vi "Aggiorna colori caselle VACON.vi"(7 "id":i32, 10 "Letture inverter":T1, 11 "Test settings":refnum<vi>) -> ()   [LabVIEW 2019]
uses:
  Letture inverter.ctl
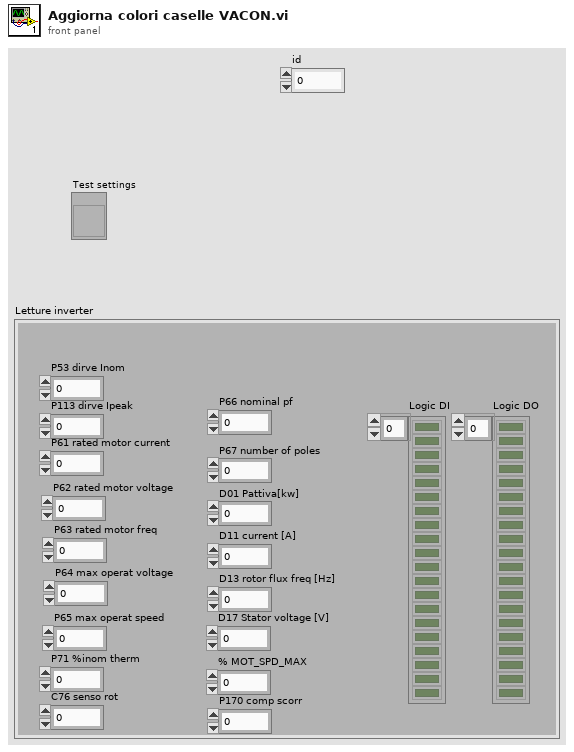
[diagram p1: front panel]
types:
  T1 = typedef "Letture inverter.ctl" = cluster{"P61 rated motor current":dbl, "P62 rated motor voltage":dbl, "P63 rated motor freq":dbl, "P64 max operat voltage":dbl, "P65 max operat speed":dbl, "P66 nominal pf":dbl, "P67 number of poles":dbl, "D01 Pattiva[kw]":dbl, "D11 current [A]":dbl, "D13 rotor flux freq [Hz]":dbl, "D17 Stator voltage [V]":dbl, "% MOT_SPD_MAX":dbl, "Logic DI":bool[], "Logic DO":bool[], "P71 %inom therm":dbl, "P53 dirve Inom":dbl, "P113 dirve Ipeak":dbl, "C76 senso rot":dbl, "P170 comp scorr":dbl}
  T2 = typedef "Parametri inverter.ctl" = cluster{"Vn [V]":dbl, "Fn [Hz]":dbl, "CosFi":dbl, "Imax [%Inom]":dbl, "#poles":dbl, "Inom [A]":dbl, "Senso rotazione":enum16{"CW", "CCW"}, "RPM nom":dbl, "Fmax[Hz]":dbl}
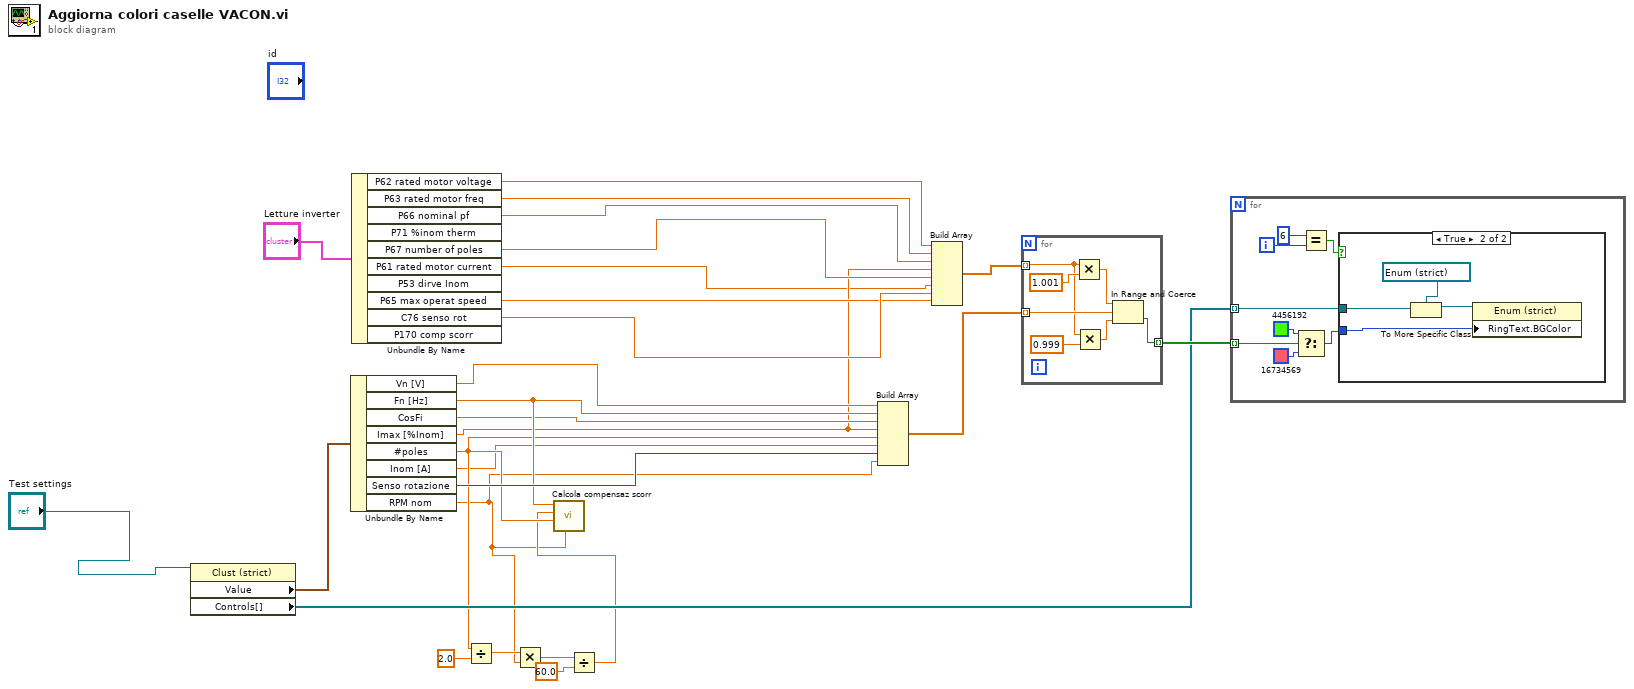
[diagram p0: block diagram]
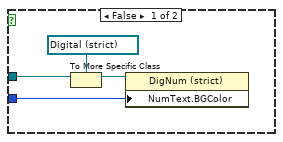
[diagram p2: hidden frame]
diagram:
  n1 = property class="Clust (strict)"(reference="Test settings") -> ("Value"=w21:T2, "Controls[]"=w22:refnum<vi>[])  [unwired: 1 in, 2 out]
  n2 = Unbundle By Name(w21) -> ("Vn [V]"=w5:dbl, "Fn [Hz]"=w16:dbl, "CosFi"=w15:dbl, "Imax [%Inom]"=w4:dbl, "#poles"=w10:dbl, "Inom [A]"=w2:dbl, "Senso rotazione"=w17:enum16{"CW", "CCW"}, "RPM nom"=w7:dbl)
  n3 = Unbundle By Name("Letture inverter") -> ("P62 rated motor voltage"=w26:dbl, "P63 rated motor freq"=w25:dbl, "P66 nominal pf"=w8:dbl, "P67 number of poles"=w24:dbl, "P61 rated motor current"=w3:dbl, "P65 max operat speed"=w6:dbl, "C76 senso rot"=w18:dbl)  [unwired: 3 out]
  n4 = Divide(x=w10, y=2.0) -> (x/y=w13:dbl)
  n5 = Multiply(x=w13, y=w7) -> (x*y=w12:dbl)
  n6 = Divide(x=w12, y=60.0) -> (x/y=w9:dbl)
  n7 = call "Calcola compensaz scorr.vi"("RPM nom"=w7, "#poles"=w10, "Fmax [Hz]"=w9, "Fn [Hz]"=w16) -> ()  [unwired: 7 in, 1 out]
  n8 = Build Array(w5, w16, w15, w4, w10, w2, w17, w7) -> (w27:dbl[])
  n9 = Build Array(w26, w25, w8, w4, w24, w3, w18, w6) -> (w19:dbl[])
  n10 = for {
    tunnel: w19 -> [w31] mode=indexing
    tunnel: w27 -> [w34] mode=indexing
    tunnel: [w28] -> w23 mode=indexing
    n11 = Multiply(x=w31, y=1.001) -> (x*y=w32:dbl)
    n12 = Multiply(x=w31, y=0.999) -> (x*y=w29:dbl)
    n13 = In Range and Coerce(upper limit=w32, x=w34, lower limit=w29) -> (In Range?=w28:bool)  [unwired: 1 out]
  }
  n14 = for {
    tunnel: w22 -> [w42] mode=indexing
    tunnel: w23 -> [w41] mode=indexing
    i -> [w37]
    n15 = Select(t=u32 4456192, s=w41, f=u32 16734569) -> (s? t:f=w38:u32)
    n16 = Equal?(x=6, y=w37) -> (x = y?=w35:bool)
    n17 = case shown="True" w35 {
      tunnel: w42 -> [w46 w49]
      tunnel: w38 -> [w45 w48]
      frame False {
        n18 = To More Specific Class(target class=refnum<vi> refnum ("Vn [V]"), reference=w46) -> (specific class reference=w44:refnum<vi>)  [unwired: 1 in, 1 out]
        n19 = property class="DigNum (strict)"(reference=w44, "NumText.BGColor"=w45) -> ()  [unwired: 1 in, 2 out]
      }
      frame True {
        n20 = To More Specific Class(target class=refnum<vi> refnum ("Senso rotazione"), reference=w49) -> (specific class reference=w50:refnum<vi>)  [unwired: 1 in, 1 out]
        n21 = property class="Enum (strict)"(reference=w50, "RingText.BGColor"=w48) -> ()  [unwired: 1 in, 2 out]
      }
    }
  }
